vi "Valve Test.vi"() -> ()   [LabVIEW 2011]
uses:
  <vilib>/DAQmx/write.llb/DAQmx Write (Digital 1D Bool 1Chan 1Samp).vi
  <vilib>/DAQmx/create/channels.llb/DAQmx Create Virtual Channel.vi
  <vilib>/DAQmx/miscellaneous.llb/DAQmx Fill In Error Info.vi
panel:
  in  "Period (s)":dbl=0.5 min=0.5 max=30.0
  in  "Duty Cycle":dbl=0.001 min=0.001 max=0.999
  in  "Valve Status":bool[](array[boolean])
  in  "stop":bool
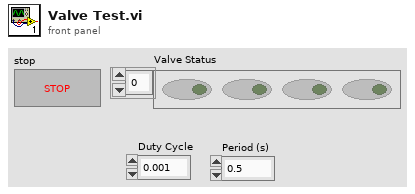
[diagram p1: front panel]
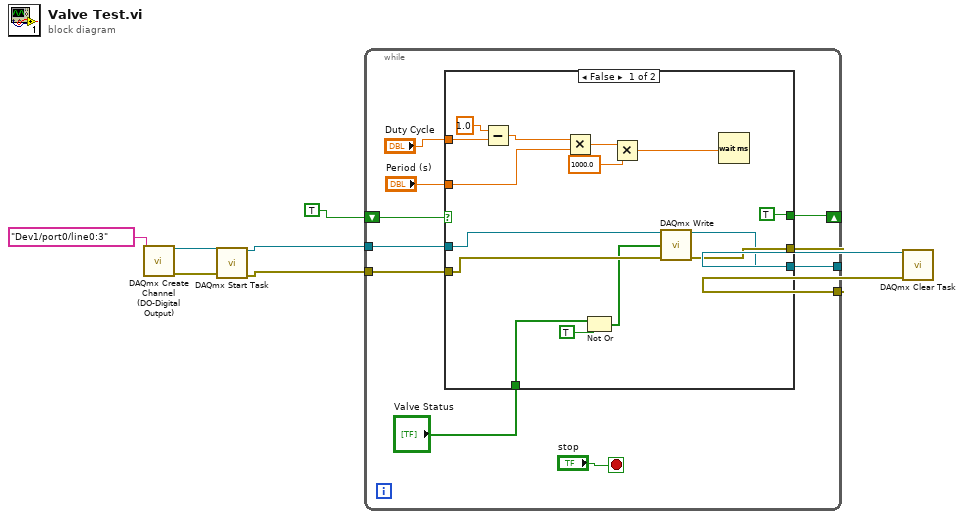
[diagram p0: block diagram]
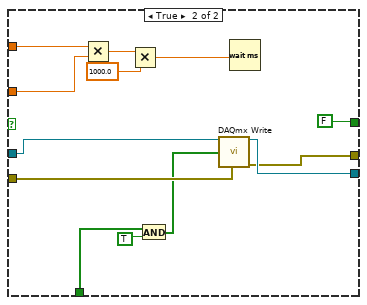
[diagram p2: hidden frame]
diagram:
  n1 = call-poly <vilib>:"DAQmx Create Channel (DO-Digital Output).vi"("lines"=tag "Dev1/port0/line0:3") -> ("task out"=w7:refnum<k21>, "error out"=w6:errorcluster)  [unwired: 13 in]
  n2 = call <vilib>:"DAQmx Start Task.vi"("task/channels in"=w7, "error in"=w6) -> ("task out"=w5:refnum<k21>, "error out"=w4:errorcluster)  [unwired: 12 in]
  n3 = while {
    tunnel: w5 -> [w17]
    tunnel: w4 -> [w16]
    tunnel: [w15] -> w3
    tunnel: [w14] -> w2
    shift-right: [w11] -> _
    shift-left: TRUE -> [w12]
    stop <- "stop" stop-if-true
    n4 = case shown="False" w12 {
      tunnel: w17 -> [w30 w46]
      tunnel: w16 -> [w29 w45]
      tunnel: [w27 w44] -> w15
      tunnel: [w28 w43] -> w14
      tunnel: "Valve Status" -> [w19 w35]
      tunnel: [TRUE FALSE] -> w11
      tunnel: "Duty Cycle" -> [w25 w41]
      tunnel: "Period (s)" -> [w31 w40]
      frame False {
        n5 = Subtract(x=1.0, y=w25) -> (x-y=w23:dbl)
        n6 = Multiply(x=w23, y=w31) -> (x*y=w32:dbl)
        n7 = Not Or(1:TRUE, 2:w19) -> (0:w20:bool[])
        n8 = Multiply(x=w32, y=1000.0) -> (x*y=w22:dbl)
        n9 = call-poly <vilib>:"DAQmx Write.vi"("task/channels in"=w30, "data"=w20, "error in"=w29) -> ("task out"=w27:refnum<k21>, "error out"=w28:errorcluster)  [unwired: 10 in, 1 out]
        n10 = Wait (ms)(milliseconds to wait=w22) -> ()  [unwired: 1 out]
      }
      frame True {
        n11 = Multiply(x=w41, y=w40) -> (x*y=w39:dbl)
        n12 = Multiply(x=w39, y=1000.0) -> (x*y=w37:dbl)
        n13 = And(x=w35, y=TRUE) -> (x .and. y?=w36:bool[])
        n14 = call-poly <vilib>:"DAQmx Write.vi"("task/channels in"=w46, "data"=w36, "error in"=w45) -> ("task out"=w44:refnum<k21>, "error out"=w43:errorcluster)  [unwired: 10 in, 1 out]
        n15 = Wait (ms)(milliseconds to wait=w37) -> ()  [unwired: 1 out]
      }
    }
  }
  n16 = call <vilib>:"DAQmx Clear Task.vi"("task in"=w3, "error in"=w2) -> ()  [unwired: 13 in, 1 out]
